vi "MapPositionSend.vi"(8 "error in (no error)":errorcluster caption="错误输入（无错误）", 10 "MapPosition":T1, 11 "States.lvlib:Localize.lvclass":refnum<class "Localize.lvclass">) -> (0 "error out":errorcluster caption="错误输出", 3 "Process State out":refnum<class "State Actor.lvclass">)   [LabVIEW 2014, in "States.lvlib" / "Localize.lvclass"]
uses:
  Localize.lvclass
  <vilib>/NI/Actors/State Actor/State Actor/State Actor.lvclass
  ctl/Point.ctl
  <vilib>/ActorFramework/Message Enqueuer/Message Enqueuer.lvclass/Message Enqueuer.ctl
  <vilib>/ActorFramework/Message Enqueuer/Enqueue.vi
  <vilib>/ActorFramework/Message Priority Queue/Priority Enqueue.vi
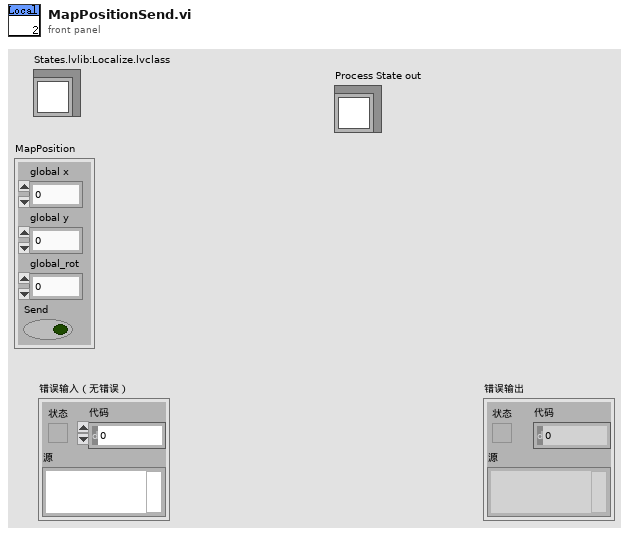
[diagram p1: front panel]
types:
  T1 = cluster{"global x":dbl, "global y":dbl, "global_rot":dbl, "Send":bool}
  T2 = typedef "Point.ctl" = cluster{"x":dbl, "y":dbl, "z":dbl}
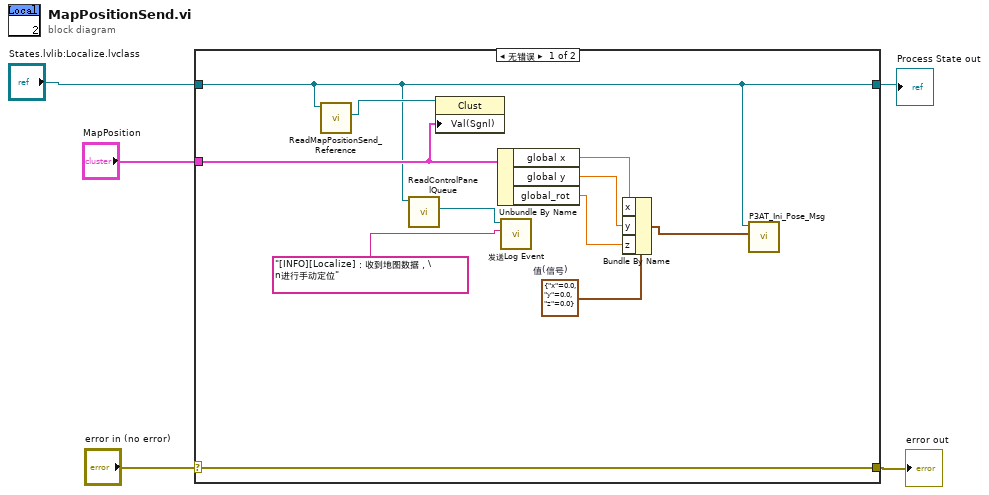
[diagram p0: block diagram]
diagram:
  n1 = case shown="无错误" "error in (no error)" {
    selector: "error in (no error)" -> [w16 w17]
    tunnel: [w16 w17] -> w4
    tunnel: [w7 w18] -> w2
    tunnel: "States.lvlib:Localize.lvclass" -> [w7 w18]
    tunnel: "MapPosition" -> [w11 _]
    frame No Error {
      w12 = T2 {"x"=0.0, "y"=0.0, "z"=0.0}  # 值(信号)
      n2 = call-dynamic "ReadMapPositionSend_Reference.vi"("CoordinatorState输入"=w7) -> ("MapPositionSend_Reference"=w13:refnum<vi>)  [unwired: 8 in, 2 out]
      n3 = call-dynamic "ReadControlPanelQueue.vi"("CoordinatorState输入"=w7) -> ("操作者框架:消息待入队列"=w15:refnum<class "Message Enqueuer.lvclass">)  [unwired: 8 in, 2 out]
      n4 = property class="Clust"(reference=w13, "Val(Sgnl)"=w11) -> ()  [unwired: 1 in, 2 out]
      n5 = Unbundle By Name(w11) -> ("global x"=w10:dbl, "global y"=w9:dbl, "global_rot"=w8:dbl)
      n6 = call "发送Log Event.vi"("Event Text"="[INFO][Localize]：收到地图数据，\n进行手动定位", "消息待入队列"=w15) -> ()  [unwired: 8 in, 2 out]
      n7 = Bundle By Name(cluster=w12, "x"=w10, "y"=w9, "z"=w8) -> (w6:T2)
      n8 = call-dynamic "P3AT_Ini_Pose_Msg.vi"("值(信号)"=w6, "States.lvlib:Localize.lvclass"=w7) -> ()  [unwired: 8 in, 2 out]
    }
    frame Error {
    }
  }
  "error out" <- w4
  "Process State out" <- w2
